vi "LX_H1.vi"(0 "datain":string[](array[string])=["备注", "负载通道", "负载地址", "延时时间", "output max", "output min", "量测类型", "待测物板号"], 5 "HW CH Number":i32=4, 7 "Setup":string) -> (4 "REPORT INDECATE":string[][](array[string])=[["微安测试", "", "", "", ""], ["微安量测", "4", "0.000", "0.1", "NG"], ["微安量测", "4", "0.000", "0.1", "NG"], ["微安量测", "4", "0.000", "0.1", "NG"], ["微安量测", "4", "0.000", "0.1", "NG"]], 6 "ROW HEAD":string[](array[string]), 8 "PF":string[](array[string]), 10 "testData":string[](array[string]), 14 "数组":bool[](array[boolean]), 15 "Array":string[](array[string]))   [LabVIEW 2018]
uses:
  Subvi/Global.vi
panel:
  out "子数组":string[](array[string])
  out "Lx Result":sgl[][](array[numeric]) format="%#_6f"
  out "测试板数":i32=4
  # "[VoltageTest]\nExt.Name =2222222222;\nAddress =1;\nDelay Time =1;\nMAX.Spec =*;\nMin.Spec =2;\nTest Type =;\nRelayH_8Bit =0,0,0,0;\nRelayL_8Bit =0,0,0,0;\nStart board number =1;#"
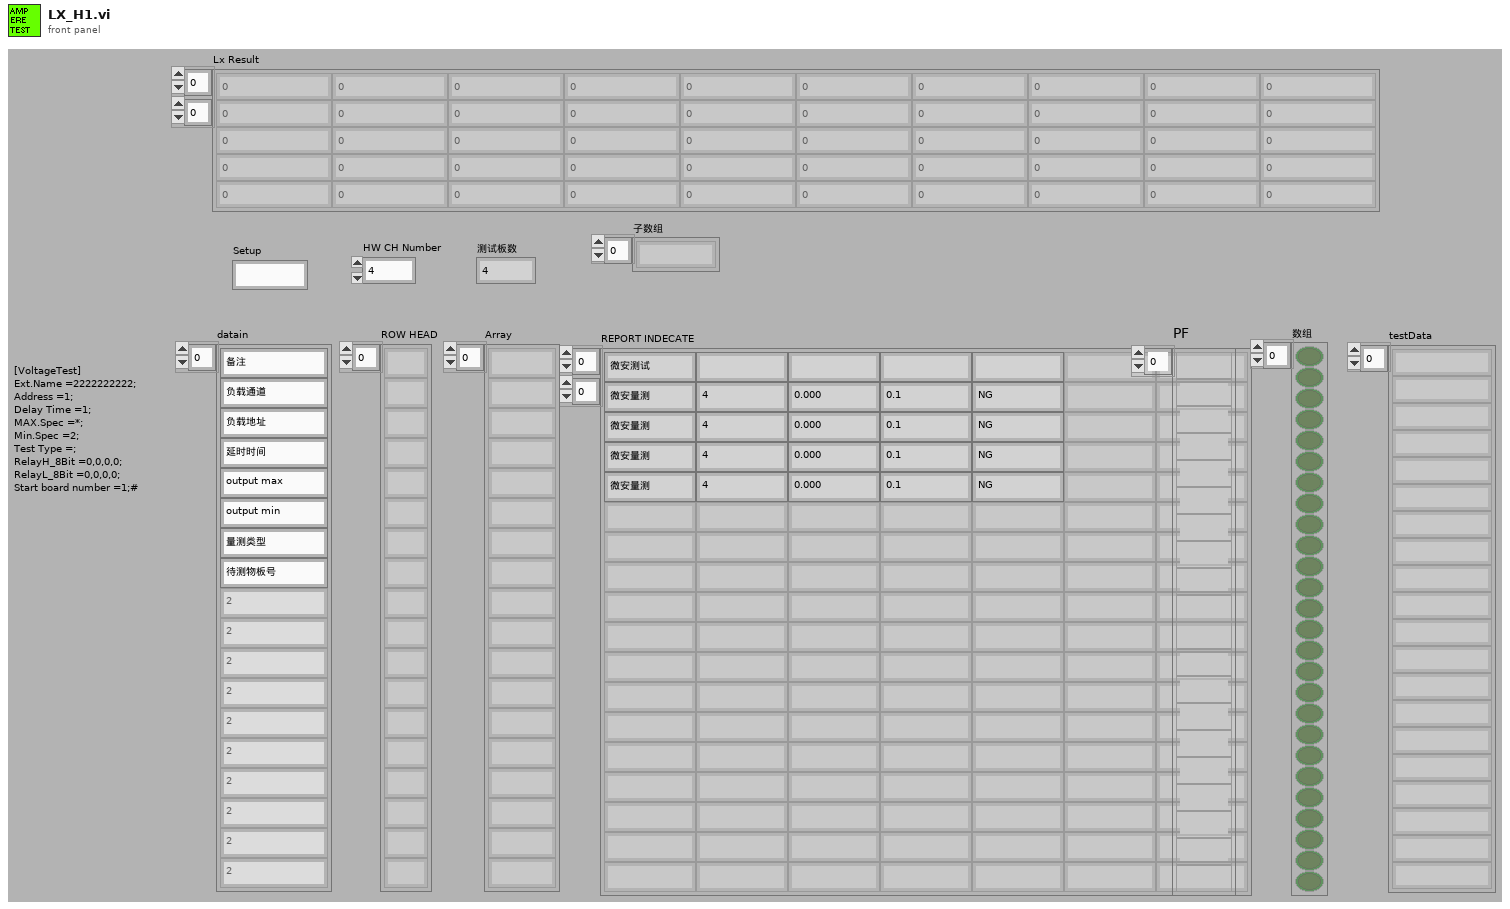
[diagram p1: front panel]
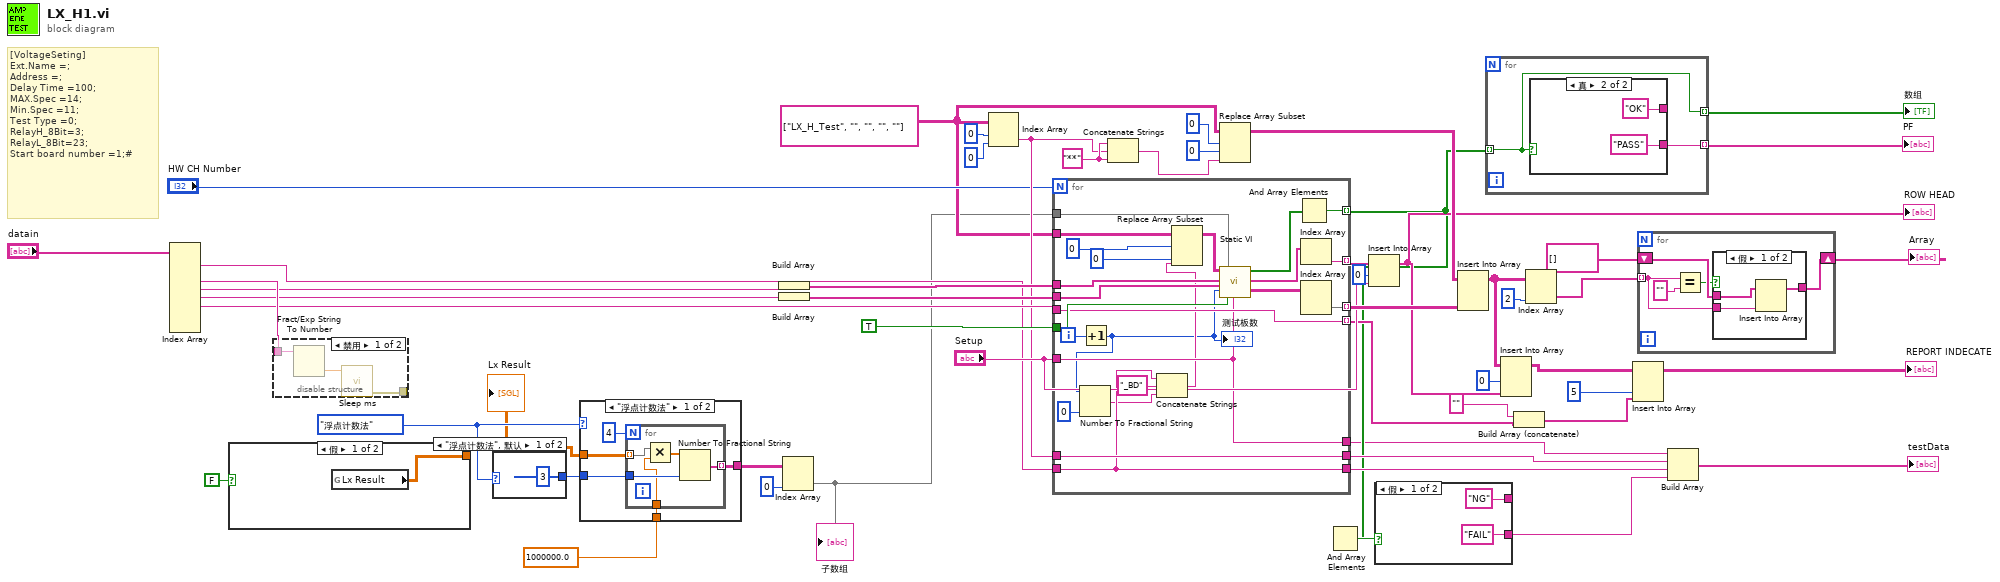
[diagram p0: block diagram]
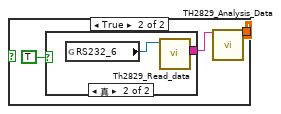
[diagram p2: hidden frame]
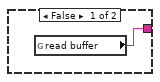
[diagram p3: hidden frame]
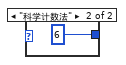
[diagram p4: hidden frame]
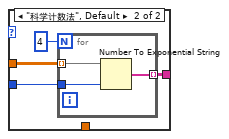
[diagram p5: hidden frame]
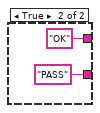
[diagram p7: hidden frame]
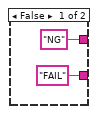
[diagram p8: hidden frame]
diagram:
  w6 = enum16{"浮点计数法", "科学计数法"}."浮点计数法" ("显示格式")
  w9 = string[][] [["LX_H_Test", "", "", "", ""]]
  w44 = "**" ("字符串")
  # "[VoltageSeting]\nExt.Name =;\nAddress =;\nDelay Time =100;\nMAX.Spec =14;\nMin.Spec =11;\nTest Type =0;\nRelayH_8Bit=3;\nRelayL_8Bit=23;\nStart board number =1;#"
  n1 = Index Array(array="datain") -> (element #1=w10:string, element #3=w47:string, element #4=w40:string, element #5=w39:string, element #6=w27:string)  [unwired: 9 in, 4 out]
  n2 = case shown="假" FALSE {
    tunnel: [w54 w55] -> w3
    frame False {
      n3 = global read "Global.vi" "Lx Result"() -> (w54:sgl[][])
    }
    frame True {
      n4 = case shown="真" TRUE {
        tunnel: [w58 w60] -> w56
        frame False {
          n5 = global read "Global.vi" "read buffer"() -> (w58:string)
        }
        frame True {
          n6 = global read "Global.vi" "RS232_6"() -> (w59:refnum<visa-resource-name>)
          n7 = call "Th2829_Read_data.vi"("VISA资源名称"=w59) -> ("读取缓冲区"=w60:string)  [unwired: 9 in, 1 out]
        }
      }
      n8 = call "TH2829_Analysis_Data.vi"("字符串"=w56) -> ("Lx Result"=w55:sgl[][])  [unwired: 15 in, 3 out]
    }
  }
  "Lx Result" <- w3
  n9 = disable-structure shown="禁用" {
    disable-tunnel: w47 -> [w63 _]
    disable-tunnel: [w62 _] -> _
    frame Disabled {
      n10 = Fract/Exp String To Number(string=w63) -> (number=w61:dbl)  [unwired: 3 in, 1 out]
      n11 = call "Sleep ms.vi"("等待时间（毫秒）"=w61) -> ("error out"=w62:errorcluster)  [unwired: 10 in]
    }
    frame Enabled {
    }
  }
  n12 = case shown="\"浮点计数法\", 默认" w6 {
    tunnel: [i16 3 ("精度(6)") i16 6 ("精度(6)")] -> w5
    frame "浮点计数法", Default {
    }
    frame "科学计数法" {
    }
  }
  n13 = case shown="\"浮点计数法\"" w6 {
    tunnel: w3 -> [w69 w78]
    tunnel: [w68 w77] -> w7
    tunnel: w5 -> [w67 w76]
    tunnel: 1000000.0 -> [w66 _]
    frame "浮点计数法" {
      n14 = for {
        N: 4 -> [_]
        tunnel: w69 -> [w72] mode=indexing
        tunnel: [w75] -> w68 mode=indexing
        tunnel: w67 -> [w74]
        tunnel: w66 -> [w71]
        n15 = Multiply(x=w72, y=w71) -> (x*y=w73:dbl[])
        n16 = Number To Fractional String(number=w73, precision (6)=w74) -> (F-format string=w75:string[])  [unwired: 2 in]
      }
    }
    frame "科学计数法", Default {
      n17 = for {
        N: 4 -> [_]
        tunnel: w78 -> [w82] mode=indexing
        tunnel: [w81] -> w77 mode=indexing
        tunnel: w76 -> [w80]
        n18 = Number To Exponential String(number=w82, precision (6)=w80) -> (E-format string=w81:string[])  [unwired: 2 in]
      }
    }
  }
  n19 = Build Array(w40) -> (w38:string[])
  n20 = Build Array(w39) -> (w37:string[])
  n21 = Index Array(array=w7, index (col)=0 ("禁用的索引 (列)")) -> (element=w4:string[])  [unwired: 1 in]
  "子数组" <- w4
  n22 = Index Array(array=w9, index (row)=0 ("索引 (行)"), index (col)=0 ("禁用的索引 (列)")) -> (element=w20:string)
  n23 = for {
    N: "HW CH Number" -> [_]
    tunnel: w4 -> [w106]
    tunnel: w38 -> [w105]
    tunnel: w37 -> [w104]
    tunnel: "Setup" -> [w94]
    tunnel: TRUE -> [w102]
    tunnel: [w101] -> w16 mode=indexing
    tunnel: [w99] -> w33 mode=indexing
    tunnel: [w97] -> w34 mode=indexing
    tunnel: w27 -> [w96]
    tunnel: [w96] -> w23 mode=indexing
    tunnel: w20 -> [w95]
    tunnel: [w95] -> w19
    tunnel: w10 -> [w86]
    tunnel: [w86] -> w18
    tunnel: [w94] -> w13
    tunnel: w9 -> [w92]
    i -> [w89]
    n24 = Increment(x=w89) -> (x+1=w83:i32)
    "测试板数" <- w83
    n25 = Number To Fractional String(number=w83, precision (6)=i16 0 ("精度(6)")) -> (F-format string=w85:string)  [unwired: 2 in]
    n26 = Concatenate Strings(w86, "_BD" ("字符串"), w85) -> (w84:string)
    n27 = Replace Array Subset(array=w92, new element=w84, index (row)=0 ("索引 (行)"), index (col)=0 ("禁用的索引 (列)")) -> (w91:string[][])
    n28 = call "Static VI.vi"("添加的数组"=w91, "Max"=w105, "Min"=w104, "板数"=w83, "INPUTSTRING"=w106, "是否为字符串对比"=w102, "SQ"=w94) -> ("P/F"=w103:bool[], "SQ out"=w100:string[], "arrauy out"=w98:string[][])  [unwired: 9 in, 1 out]
    n29 = And Array Elements(Boolean array=w103) -> (logical AND=w101:bool)
    n30 = Index Array(array=w100) -> (element=w99:string)  [unwired: 1 in]
    n31 = Index Array(array=w98) -> (element=w97:string[])  [unwired: 2 in]
  }
  n32 = Concatenate Strings(w44, w20, w44) -> (w41:string)
  n33 = Replace Array Subset(array=w9, new element=w41, index (row)=0 ("索引 (行)"), index (col)=0 ("禁用的索引 (列)")) -> (w35:string[][])
  n34 = And Array Elements(Boolean array=w16) -> (logical AND=w17:bool)
  n35 = Insert Into Array(array=w33, index=0 ("索引"), new element="Setup") -> (w29:string[])
  "ROW HEAD" <- w29
  n36 = case shown="假" w17 {
    tunnel: ["NG" "OK"] -> _
    tunnel: ["FAIL" "PASS"] -> w15
    frame False {
    }
    frame True {
    }
  }
  n37 = Insert Into Array ("数组插入")(array=w35, new element=w34) -> (w30:string[][])  [unwired: 2 in]
  n38 = for {
    tunnel: w16 -> [w111] mode=indexing
    tunnel: [w112] -> w49 mode=indexing
    tunnel: [w111] -> w12 mode=indexing
    n39 = case shown="真" w111 {
      tunnel: ["NG" "OK"] -> _
      tunnel: ["FAIL" "PASS"] -> w112
      frame False {
      }
      frame True {
      }
    }
  }
  "PF" <- w49
  "数组" <- w12
  n40 = Insert Into Array(array=w30, index (col)=0 ("禁用的索引 (列)"), new element=w29) -> (w25:string[][])  [unwired: 1 in]
  n41 = Build Array (concatenate)("" ("字符串"), w23) -> (w21:string[])
  n42 = Index Array(array=w30, index (col)=2 ("禁用的索引 (列)")) -> (element=w51:string[])  [unwired: 1 in]
  n43 = Insert Into Array(array=w25, index (col)=5 ("禁用的索引 (列)"), new element=w21) -> (→"REPORT INDECATE":string[][])  [unwired: 1 in]
  n44 = for {
    tunnel: w51 -> [w117] mode=indexing
    shift-right: [w118] -> w50
    shift-left: string[] [] ("Array") -> [w121]
    n45 = Equal?(x=w117, y="") -> (x = y?=w119:bool)
    n46 = case shown="假" w119 {
      tunnel: w121 -> [w124 w125]
      tunnel: [w123 w125] -> w118
      tunnel: w117 -> [w122 _]
      frame False {
        n47 = Insert Into Array(array=w124, new element=w122) -> (w123:string[])  [unwired: 1 in]
      }
      frame True {
      }
    }
  }
  "Array" <- w50
  n48 = Build Array(w13, w19, w18, w15) -> (→"testData":string[])
